vi "setUserEvents.vi"(10 "UserEvents":refnum<class "UserEvents.lvclass">, 11 "Model in":refnum<class "Model.lvclass">) -> (3 "Model out":refnum<class "Model.lvclass">)   [LabVIEW 2016, in "Model.lvclass"]
uses:
  Model.lvclass
  UserEvents/UserEvents.lvclass
  Model.lvclass/Model.ctl
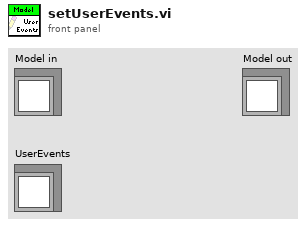
[diagram p1: front panel]
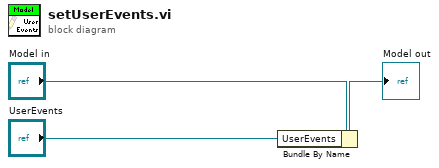
[diagram p0: block diagram]
diagram:
  n1 = Bundle By Name(cluster="Model in", "UserEvents"="UserEvents") -> (→"Model out":refnum<class "Model.lvclass">)
